vi "vibrations.vi"() -> ()   [LabVIEW 2024]
uses:
  <vilib>/express/express analysis/Spectral/XNode/ExpressSpectralMeasurementsBlockNode.xnode
  <vilib>/express/express analysis/Spectral/Block/exnSpectralBlock spectral measurements RMS poly.vi
  <vilib>/express/express analysis/Spectral/Block/exnSpectralBlock spectral measurements RMS WFM.vi
panel:
  out "Waveform Graph":waveform(dbl)(graph)
  in  "Array":T1(array[cluster]) {"Amplitude" scale=0.0..10.0; "Phase" scale=0.0..180.0; "Frequency" scale=0.0..100.0}
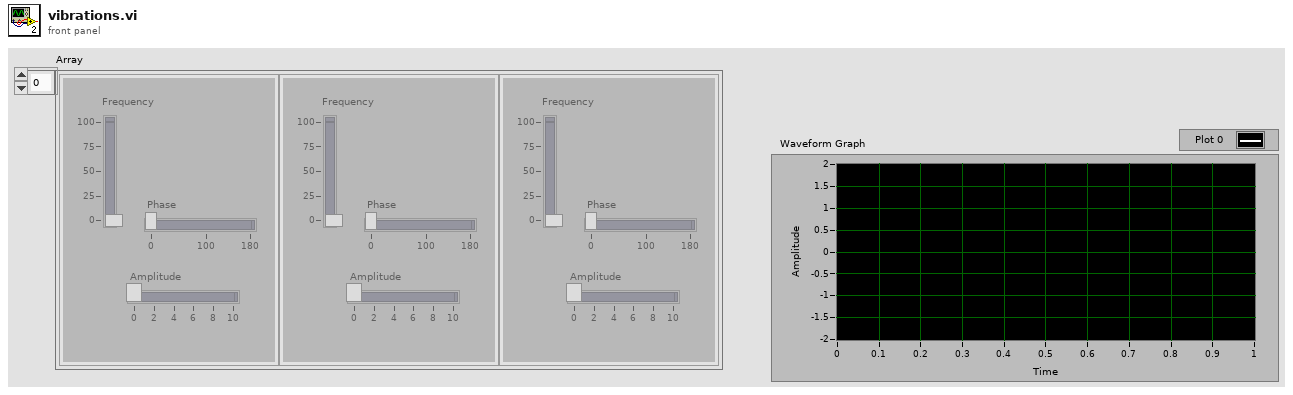
[diagram p1: front panel]
types:
  T1 = cluster{"Frequency":dbl, "Phase":dbl, "Amplitude":dbl}[]
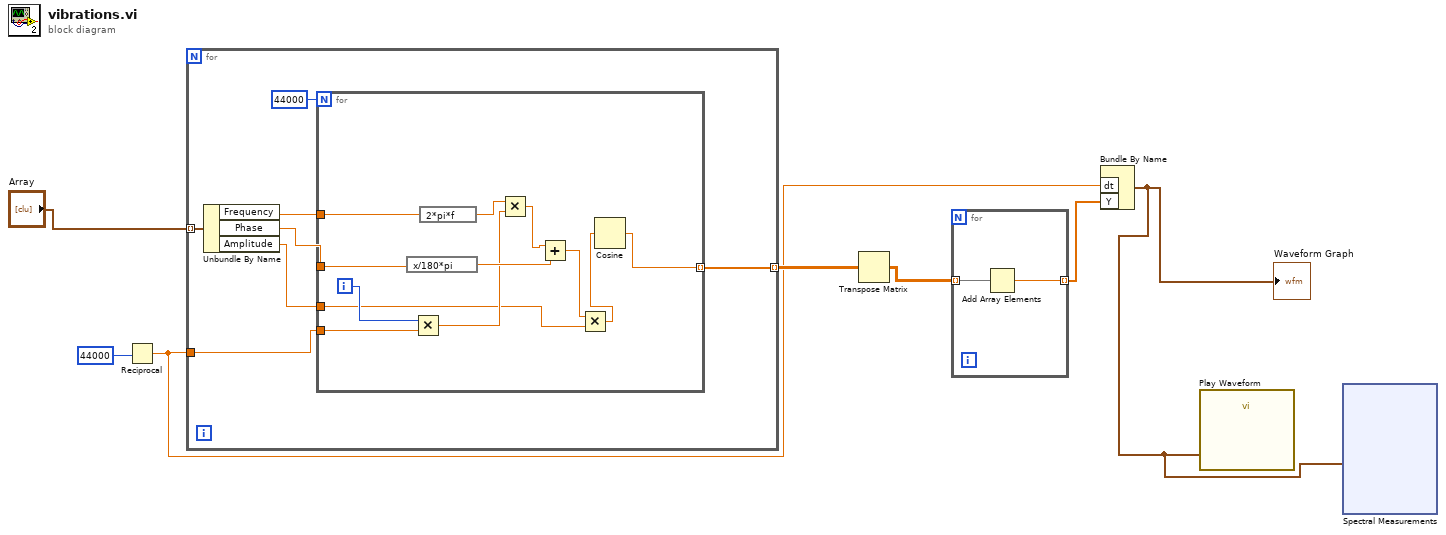
[diagram p0: block diagram]
diagram:
  n1 = Reciprocal(x=44000) -> (1/x=w2:dbl)
  n2 = for {
    tunnel: w2 -> [w13]
    tunnel: [w12] -> w6 mode=indexing
    tunnel: "Array" -> [w9] mode=indexing
    n3 = Unbundle By Name(w9) -> ("Frequency"=w11:dbl, "Phase"=w10:dbl, "Amplitude"=w8:dbl)
    n4 = for {
      N: 44000 -> [_]
      tunnel: w13 -> [w21]
      tunnel: w11 -> [w20]
      tunnel: w10 -> [w19]
      tunnel: [w18] -> w12 mode=indexing
      tunnel: w8 -> [w17]
      i -> [w24]
      n5 = expression code="x/180*pi"(w19) -> (w26:dbl)
      n6 = Multiply(x=w24, y=w21) -> (x*y=w23:dbl)
      n7 = expression code="2*pi*f"(w20) -> (w25:dbl)
      n8 = Multiply(x=w25, y=w23) -> (x*y=w22:dbl)
      n9 = Add(x=w22, y=w26) -> (x+y=w16:dbl)
      n10 = Multiply(x=w16, y=w17) -> (x*y=w15:dbl)
      n11 = Cosine(x=w15) -> (cos(x)=w18:dbl)
    }
  }
  n12 = Transpose Matrix(1:w6) -> (0:w5:dbl[][])
  n13 = for {
    tunnel: w5 -> [w28] mode=indexing
    tunnel: [w27] -> w3 mode=indexing
    n14 = Add Array Elements(numeric array=w28) -> (sum=w27:dbl)
  }
  n15 = Bundle By Name("dt"=w2, "Y"=w3) -> (w1:waveform(dbl))  [unwired: 1 in]
  "Waveform Graph" <- w1
  n16 = call "Play Waveform"("Data"=w1) -> ()  [unwired: 18 in, 1 out]
  n17 = xnode "Spectral Measurements"("Signals"=w1) -> ()  [unwired: 1 in, 3 out]
